vi "VFH Wrapper (SubVI).vi"(8 "Error In":errorcluster, 9 "Theta Actual (rad)":dbl, 10 "Goal Position (m)":dbl[](array[numeric]), 11 "Current Position (m)":dbl[](array[numeric])) -> (0 "Error Out":errorcluster, 1 "Min Speed (m/s)":dbl, 2 "Max Speed (m/s)":dbl, 3 "chosen heading (rad)":dbl)   [LabVIEW 2017]
uses:
  <vilib>/robotics/Obstacle Avoidance/Advanced Vector Field Histogram/NI_Robotics_Vector Field Histogram.lvlib
panel:
  out "chosen heading (deg)":dbl
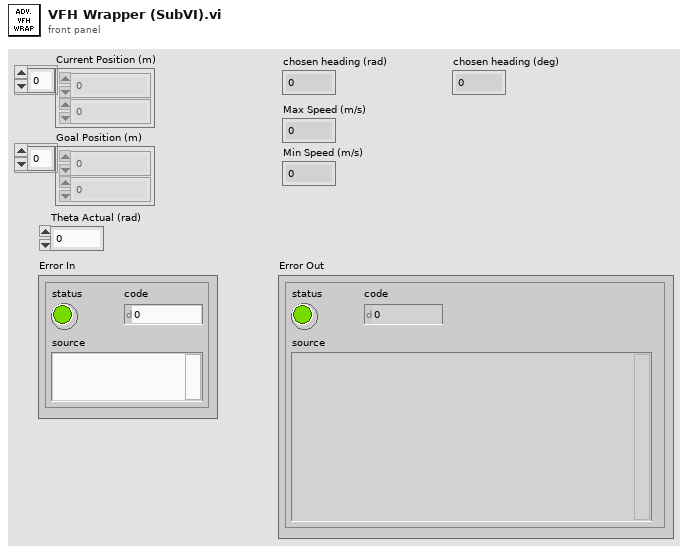
[diagram p1: front panel]
types:
  T1 = cluster{"Theta Actual (rad)":dbl, "Target Heading":dbl}
  T2 = cluster{"inner threshold distance":dbl, "inner threshold distance":dbl}
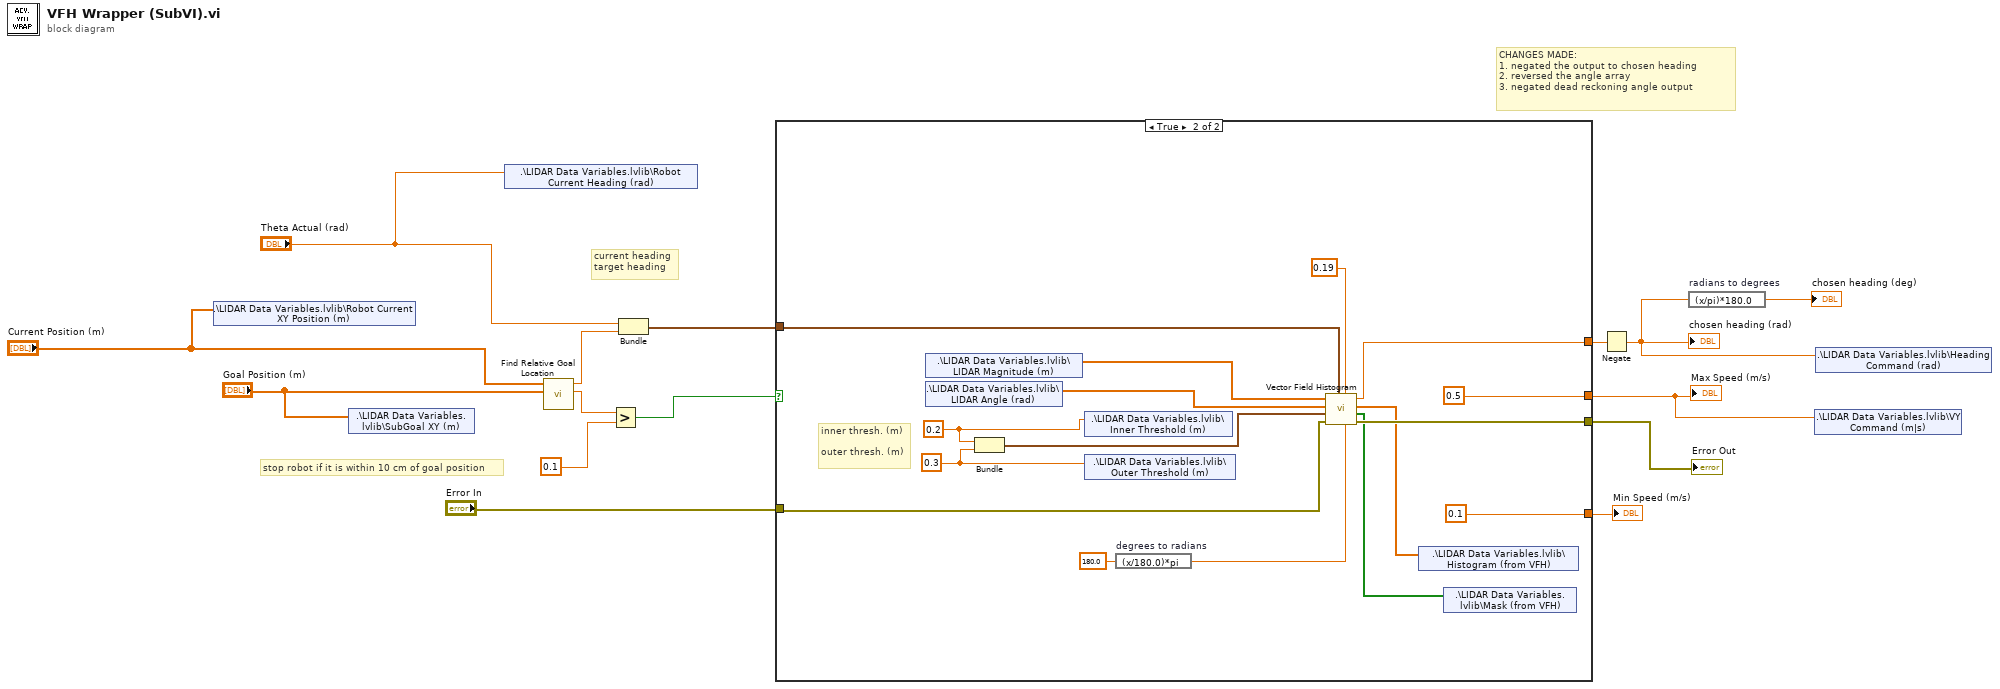
[diagram p0: block diagram]
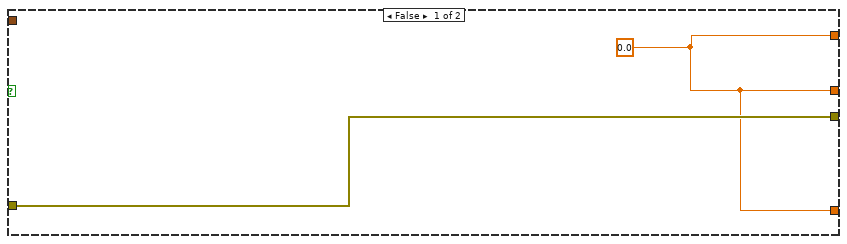
[diagram p2: hidden frame]
diagram:
  # "CHANGES MADE: \n1. negated the output to chosen heading\n2. reversed the angle array\n3. negated dead reckoning angle output"
  # "stop robot if it is within 10 cm of goal position"
  # "current heading\ntarget heading"
  n1 = shared-variable ".\\LIDAR Data Variables.lvlib\\Robot Current XY Position (m)"("Current Position (m)") -> ()  [unwired: 1 in, 1 out]
  n2 = shared-variable ".\\LIDAR Data Variables.lvlib\\SubGoal XY (m)"("Goal Position (m)") -> ()  [unwired: 1 in, 1 out]
  n3 = shared-variable ".\\LIDAR Data Variables.lvlib\\Robot Current Heading (rad)"("Theta Actual (rad)") -> ()  [unwired: 1 in, 1 out]
  n4 = call "Find Relative Goal Location.vi"("Goal Position"="Goal Position (m)", "Current Position"="Current Position (m)") -> ("Target Distance"=w14:dbl, "Target Heading"=w2:dbl)  [unwired: 8 in]
  n5 = Greater?(x=w14, y=0.1) -> (0:w12:bool)
  n6 = Bundle("Theta Actual (rad)"="Theta Actual (rad)", "Target Heading"=w2) -> (w15:T1)  [unwired: 1 in]
  n7 = case shown="True" w12 {
    tunnel: [w16 w18] -> w8
    tunnel: w15 -> [_ w32]
    tunnel: "Error In" -> [w17 w31]
    tunnel: [w17 w30] -> w10
    tunnel: [w16 0.5 ("obstacle clearance distance")] -> w7
    tunnel: [w16 0.1 ("obstacle clearance distance")] -> w1
    frame False {
      w16 = 0.0 ("chosen heading (rad)")
    }
    frame True {
      w21 = 0.3 ("inner threshold distance")
      w22 = 0.2 ("inner threshold distance")
      # "inner thresh. (m)\n\nouter thresh. (m)"
      n8 = shared-variable ".\\LIDAR Data Variables.lvlib\\LIDAR Magnitude (m)"() -> (w26:dbl[])  [unwired: 1 in, 1 out]
      n9 = shared-variable ".\\LIDAR Data Variables.lvlib\\LIDAR Angle (rad)"() -> (w25:dbl[])  [unwired: 1 in, 1 out]
      n10 = Bundle("inner threshold distance"=w22, "inner threshold distance"=w21) -> (w23:T2)  [unwired: 1 in]
      n11 = shared-variable ".\\LIDAR Data Variables.lvlib\\Inner Threshold (m)"(w22) -> ()  [unwired: 1 in, 1 out]
      n12 = shared-variable ".\\LIDAR Data Variables.lvlib\\Outer Threshold (m)"(w21) -> ()  [unwired: 1 in, 1 out]
      n13 = expression code="(x/180.0)*pi" "degrees to radians"(180.0) -> (w27:dbl)
      n14 = call <vilib>:"Vector Field Histogram.vi"("maximum heading change (rad)"=w27, "obstacle clearance distance"=0.19, "heading"=w32, "error in (no error)"=w31, "thresholds"=w23, "direction angles (rad)"=w25, "distances"=w26) -> ("error out"=w30:errorcluster, "mask"=w20:bool[], "histogram"=w24:dbl[], "chosen heading (rad)"=w18:dbl)  [unwired: 1 in]
      n15 = shared-variable ".\\LIDAR Data Variables.lvlib\\Histogram (from VFH)"(w24) -> ()  [unwired: 1 in, 1 out]
      n16 = shared-variable ".\\LIDAR Data Variables.lvlib\\Mask (from VFH)"(w20) -> ()  [unwired: 1 in, 1 out]
    }
  }
  "Error Out" <- w10
  "Max Speed (m/s)" <- w7
  "Min Speed (m/s)" <- w1
  n17 = Negate(x=w8) -> (-x=w3:dbl)
  "chosen heading (rad)" <- w3
  n18 = expression code="(x/pi)*180.0" "radians to degrees"(w3) -> (→"chosen heading (deg)":dbl)
  n19 = shared-variable ".\\LIDAR Data Variables.lvlib\\VY Command (m|s)"(w7) -> ()  [unwired: 1 in, 1 out]
  n20 = shared-variable ".\\LIDAR Data Variables.lvlib\\Heading Command (rad)"(w3) -> ()  [unwired: 1 in, 1 out]
